vi "NPC3SG Connect v10.6.0.vi"(4 "Drive Port":refnum<visa-resource-name>="COM5" caption="Visa Port") -> (0 "Success":bool, 1 "Drive Visa Name":refnum<visa-resource-name>)   [LabVIEW 2010]
uses:
  drivers/Newport NPC3SG/SubNPC3SG.llb/device variables.vi
panel:
  out "Read Error":errorcluster caption="error out" {"code" format="%x"}
  out "Connection Error":errorcluster
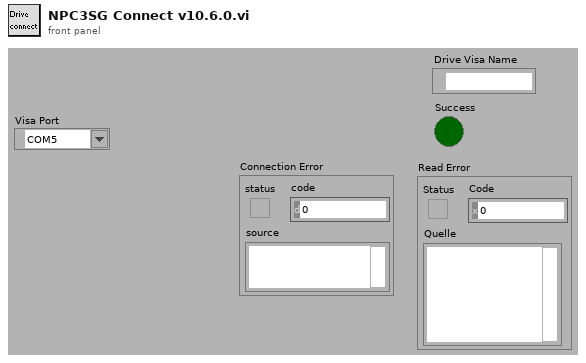
[diagram p1: front panel]
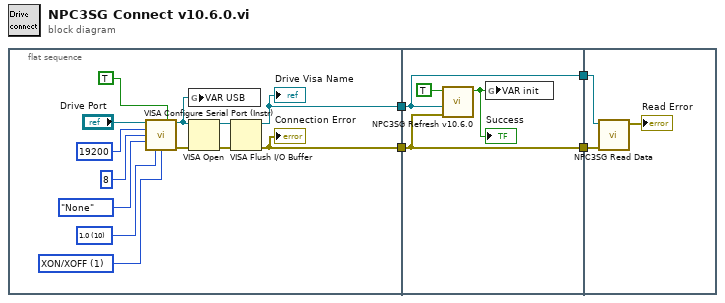
[diagram p0: block diagram]
diagram:
  n1 = flat-sequence {
    tunnel: [w7] -> w2
    tunnel: [w6] -> w1
    tunnel: w2 -> [w19]
    tunnel: w1 -> [w18]
    tunnel: [w19] -> w4
    tunnel: [w18] -> w3
    tunnel: w4 -> [w23]
    tunnel: w3 -> [w22]
    frame #0 {
      w9 = u16 1 items=["Kein", "XON/XOFF", "RTS/CTS", "XON/XOFF & RTS/CTS", "DTR/DSR", "XON/XOFF & DTR/DSR"] ("flow control (0:none)")
      w17 = u16 10 items=["1.0"=10, "1.5"=15, "2.0"=20] ("stop bits (10: 1 bit)")
      n2 = call <vilib>:"VISA Configure Serial Port (Instr).vi"("VISA resource name"="Drive Port", "Enable Termination\nChar (T)"=TRUE ("Enable Termination\nChar (T)"), "baud rate (9600)"=u32 19200, "data bits (8)"=u16 8, "parity (0:none)"=enum16{"None", "Odd", "Even", "Mark", "Space"}."None", "stop bits (10: 1 bit)"=w17, "flow control (0:none)"=w9) -> ("VISA resource name out"=w8:refnum<visa-resource-name>, "error out"=w11:errorcluster)  [unwired: 7 in]
      n3 = global write "device variables.vi" "VAR USB"(w8) -> ()
      n4 = VISA Open(error in (no error)=w11, VISA resource name=w8) -> (VISA resource name=w12:refnum<visa-resource-name>, error out=w13:errorcluster)  [unwired: 3 in]
      n5 = VISA Flush I/O Buffer(VISA resource name=w12, error in (no error)=w13) -> (VISA resource name out=w7:refnum<visa-resource-name>, error out=w6:errorcluster)  [unwired: 1 in]
      "Connection Error" <- w6
      "Drive Visa Name" <- w7
    }
    frame #1 {
      n6 = call "NPC3SG Refresh v10.6.0.vi"("error in"=w18, "VISA-Ressourcen-Name (In)"=w19, "reset all"=TRUE) -> ("init ok??"=w21:bool)  [unwired: 8 in]
      "Success" <- w21
      n7 = global write "device variables.vi" "VAR init"(w21) -> ()
    }
    frame #2 {
      n8 = call "NPC3SG Read Data.vi"("VISA resource name in"=w23, "error in"=w22) -> ("error ende"=→"Read Error":errorcluster)  [unwired: 8 in]
    }
  }
